vi "levele.vi"(7 "reset(F)":bool, 8 "Peroid(ms)":u32=5000, 9 "period(0.1s)":dbl=0.1 format="%#_13g", 11 "#Left In Q":dbl) -> (0 "s? t:f":u32, 2 "LogInQ changing Speed(#/s)":dbl, 3 "Enum":T1)   [LabVIEW 2017, in "Communicable State Machine.lvlib"]
uses:
  Communicable State Machine.lvlib
  _support/Periodic String Filter Level.ctl
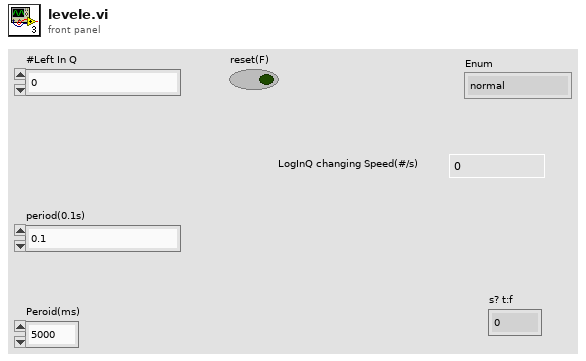
[diagram p1: front panel]
types:
  T1 = typedef "Communicable State Machine.lvlib/Periodic String Filter Level.ctl" = enum16{"normal", "L1", "L2", "L3", "L4"}
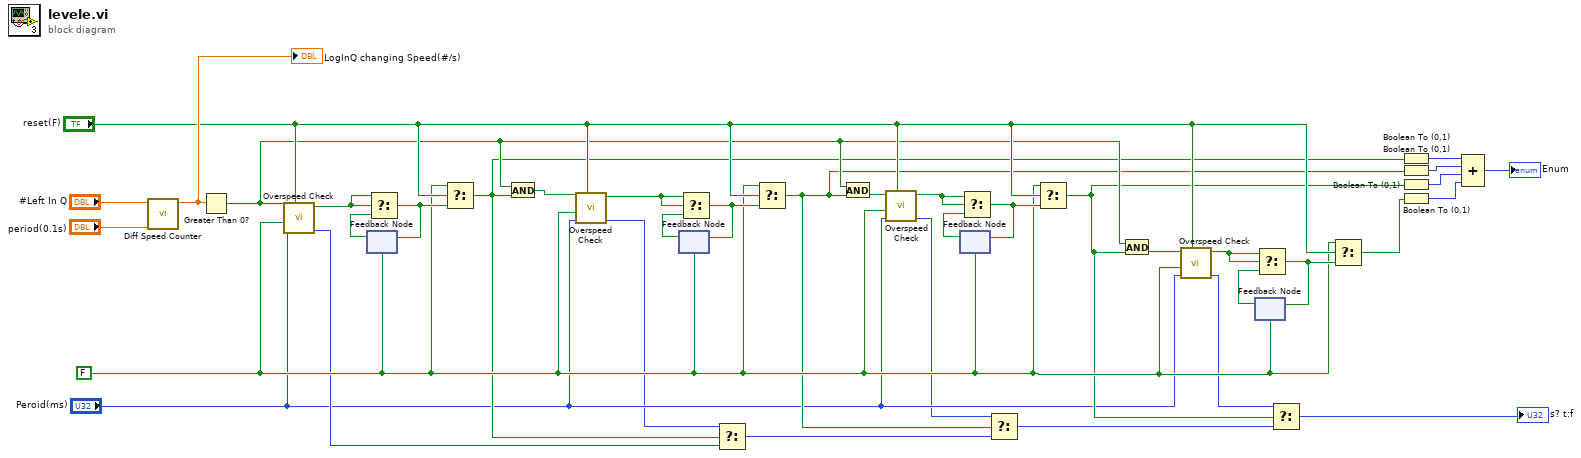
[diagram p0: block diagram]
diagram:
  w18 = FALSE ("reset value")
  n1 = call "Diff Speed Counter.vi"("period(0.1s)"="period(0.1s)", "Numeric"="#Left In Q") -> ("Speed(#/s)"=w36:dbl)  [unwired: 7 in, 2 out]
  "LogInQ changing Speed(#/s)" <- w36
  n2 = Greater Than 0?(x=w36) -> (x > 0?=w13:bool)
  n3 = call "Overspeed Check.vi"("reset(F)"="reset(F)", "Peroid(ms)"="Peroid(ms)", "reset value"=w18, "Signal"=w13) -> ("变化过去时间(ms)"=w6:u32, "signal(safe)"=w37:bool)  [unwired: 6 in]
  n4 = feedback #1(w18) -> (w38:bool)
  n5 = Select(t=w37, s=w37, f=w38) -> (s? t:f=w33:bool)
  n6 = feedback-in #1(w33) -> ()
  n7 = Select(t=w18, s="reset(F)", f=w33) -> (s? t:f=w8:bool)
  n8 = And(x=w13, y=w8) -> (x .and. y?=w16:bool)
  n9 = call "Overspeed Check.vi"("reset(F)"="reset(F)", "Peroid(ms)"="Peroid(ms)", "reset value"=w18, "Signal"=w16) -> ("变化过去时间(ms)"=w4:u32, "signal(safe)"=w30:bool)  [unwired: 6 in]
  n10 = feedback #2(w18) -> (w31:bool)
  n11 = Select(t=w30, s=w30, f=w31) -> (s? t:f=w32:bool)
  n12 = feedback-in #2(w32) -> ()
  n13 = Select(t=w4, s=w8, f=w6) -> (s? t:f=w7:u32)
  n14 = Select(t=w18, s="reset(F)", f=w32) -> (s? t:f=w12:bool)
  n15 = And(x=w13, y=w12) -> (x .and. y?=w15:bool)
  n16 = call "Overspeed Check.vi"("reset(F)"="reset(F)", "Peroid(ms)"="Peroid(ms)", "reset value"=w18, "Signal"=w15) -> ("变化过去时间(ms)"=w3:u32, "signal(safe)"=w27:bool)  [unwired: 6 in]
  n17 = feedback #3(w18) -> (w29:bool)
  n18 = Select(t=w27, s=w27, f=w29) -> (s? t:f=w28:bool)
  n19 = feedback-in #3(w28) -> ()
  n20 = Select(t=w3, s=w12, f=w7) -> (s? t:f=w10:u32)
  n21 = Select(t=w18, s="reset(F)", f=w28) -> (s? t:f=w11:bool)
  n22 = And(x=w13, y=w11) -> (x .and. y?=w14:bool)
  n23 = call "Overspeed Check.vi"("reset(F)"="reset(F)", "Peroid(ms)"="Peroid(ms)", "reset value"=w18, "Signal"=w14) -> ("变化过去时间(ms)"=w2:u32, "signal(safe)"=w22:bool)  [unwired: 6 in]
  n24 = feedback #4(w18) -> (w20:bool)
  n25 = Select(t=w22, s=w22, f=w20) -> (s? t:f=w21:bool)
  n26 = feedback-in #4(w21) -> ()
  n27 = Select(t=w2, s=w11, f=w10) -> (s? t:f=→"s? t:f":u32)
  n28 = Select(t=w18, s="reset(F)", f=w21) -> (s? t:f=w9:bool)
  n29 = Boolean To (0,1)(Boolean=w8) -> (0, 1=w26:i16)
  n30 = Boolean To (0,1)(Boolean=w12) -> (0, 1=w25:i16)
  n31 = Boolean To (0,1)(Boolean=w11) -> (0, 1=w24:i16)
  n32 = Boolean To (0,1)(Boolean=w9) -> (0, 1=w17:i16)
  n33 = Compound Arithmetic op=ADD(w26, w25, w24, w17) -> (→"Enum":i16)
